vi "Motor Safety Limits.vi"(10 "Reference Voltage in":dbl, 11 "Boolean":bool) -> (3 "Reference Voltage out":dbl)   [LabVIEW 2018]
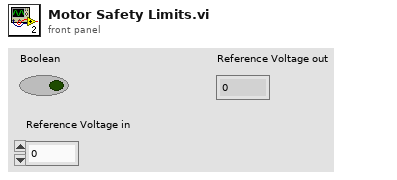
[diagram p1: front panel]
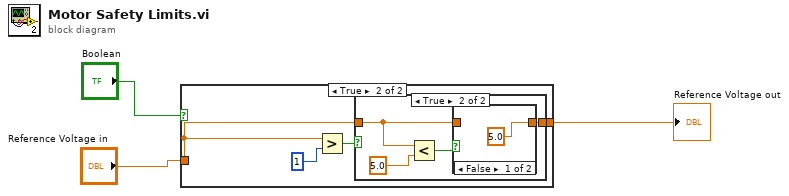
[diagram p0: block diagram]
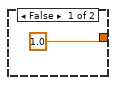
[diagram p3: hidden frame]
diagram:
  n1 = case shown="True" "Boolean" {
    tunnel: [w4 w6] -> w2
    tunnel: "Reference Voltage in" -> [w4 w5]
    frame False {
    }
    frame True {
      n2 = Greater?(x=w5, y=1) -> (0:w8:bool)
      n3 = case shown="True" w8 {
        tunnel: w5 -> [_ w11]
        tunnel: [1.0 ("y") w10] -> w6
        frame False {
        }
        frame True {
          n4 = Less?(x=w11, y=5.0) -> (x < y?=w13:bool)
          n5 = case shown="False" w13 {
            tunnel: w11 -> [_ w15]
            tunnel: [5.0 ("y") w15] -> w10
            frame False {
            }
            frame True {
            }
          }
        }
      }
    }
  }
  "Reference Voltage out" <- w2
